vi "Initialize Settings.vi"(11 "error in (no error)":errorcluster) -> (4 "Name":string, 6 "VISA resource name 2":refnum<visa-resource-name>, 15 "error out":errorcluster)   [LabVIEW 2013, in "Bioreactor.lvlib" / "Bioreactor.lvclass"]
uses:
  Bioreactor.lvclass
panel:
  in  "Bioreactor COM Port":refnum<visa-resource-name>
  in  "Bioreactor Address (HEX)":string
  in  "Button":bool
  # "Enter System Parameters"
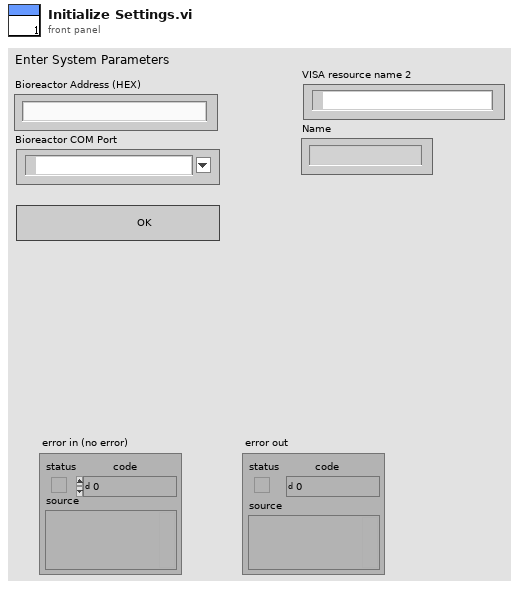
[diagram p1: front panel]
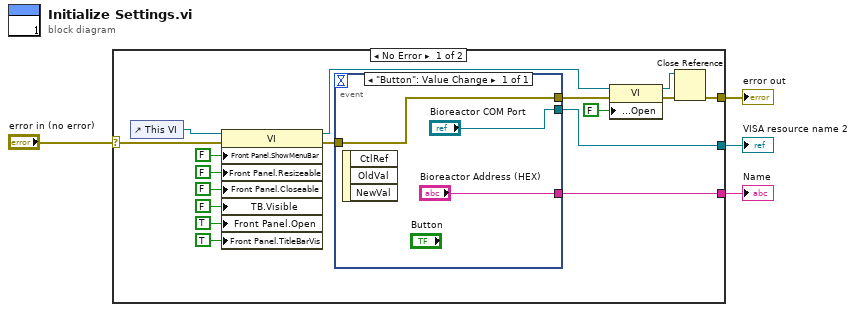
[diagram p0: block diagram]
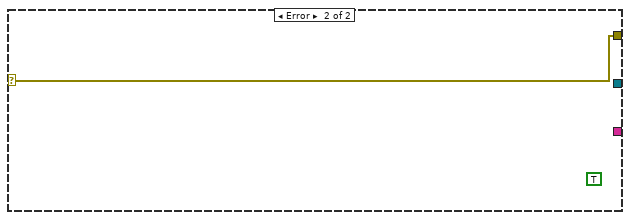
[diagram p2: hidden frame]
diagram:
  n1 = case shown="No Error" "error in (no error)" {
    selector: "error in (no error)" -> [w14 w25]
    tunnel: [w9 w25] -> w3
    tunnel: [w6 _] -> w2
    tunnel: [w5 _] -> w1
    frame No Error {
      n2 = control-ref of="This VI"() -> (w21:refnum<vi>)
      n3 = property class="VI"(reference=w21, error in=w14, "Front Panel.ShowMenuBar"=FALSE ("Front Panel Window:Show Menu Bar"), "Front Panel.Resizeable"=FALSE ("Front Panel Window:Resizable"), "Front Panel.Closeable"=FALSE ("Front Panel Window:Closeable"), "TB.Visible"=FALSE ("Tool Bar:Visible"), "Front Panel.Open"=TRUE ("Front Panel Window:Open"), "Front Panel.TitleBarVis"=TRUE ("Front Panel Window:Title Bar Visible")) -> (reference out=w8:refnum<vi>, error out=w13:errorcluster)
      n4 = event shown="[0] \"Button\": Value Change" {
        selector: _ -> [_]
        dyn-events: _ -> [_]
        timeout: _ -> [_]
        tunnel: w13 -> [w24]
        tunnel: [w24] -> w7
        tunnel: ["Bioreactor Address (HEX)"] -> w6
        tunnel: ["Bioreactor COM Port"] -> w5
        event "Button": Value Change {
          n5 = event-data() -> ()  [unwired: 1 in, 3 out]
        }
      }
      n6 = property class="VI"(reference=w8, error in=w7, "Front Panel.Open"=FALSE ("Front Panel Window:Open")) -> (reference out=w12:refnum<vi>, error out=w11:errorcluster)
      n7 = Close Reference(reference=w12, error in (no error)=w11) -> (error out=w9:errorcluster)
    }
    frame Error {
      (unwired) TRUE ("Front Panel Window:Open")
    }
  }
  "error out" <- w3
  "Name" <- w2
  "VISA resource name 2" <- w1
